vi "Edit Auton Queue Items.vi"(10 "Add?":bool, 11 "Delete?":bool) -> ()   [LabVIEW 2015]
uses:
  Robot Global Data.vi
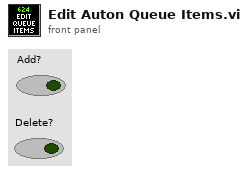
[diagram p1: front panel]
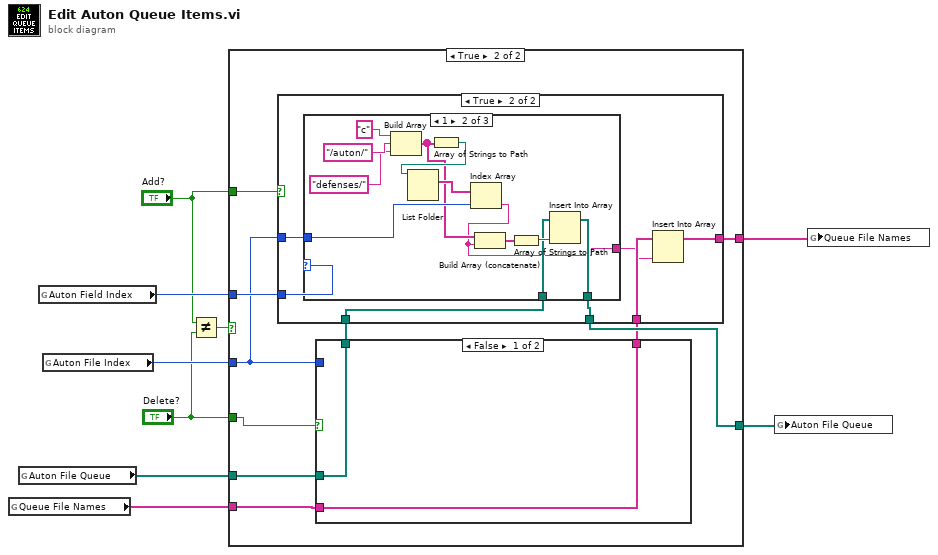
[diagram p0: block diagram]
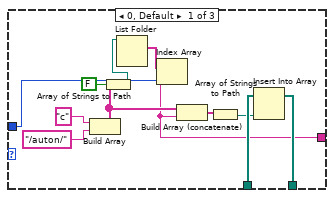
[diagram p4: hidden frame]
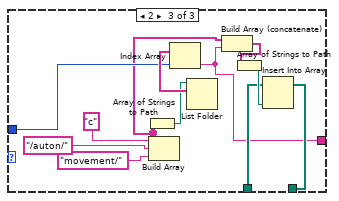
[diagram p5: hidden frame]
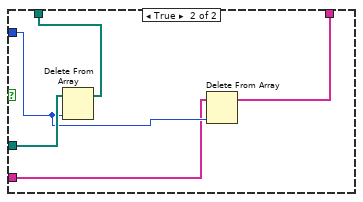
[diagram p6: hidden frame]
diagram:
  n1 = global read "Robot Global Data.vi" "Queue File Names"() -> (w2:string[])
  n2 = global read "Robot Global Data.vi" "Auton File Queue"() -> (w4:path[])
  n3 = global read "Robot Global Data.vi" "Auton Field Index"() -> (w9:i32)
  n4 = global read "Robot Global Data.vi" "Auton File Index"() -> (w8:i32)
  n5 = Not Equal?(x="Add?", y="Delete?") -> (x != y?=w5:bool)
  n6 = case shown="True" w5 {
    tunnel: "Add?" -> [_ w18]
    tunnel: "Delete?" -> [_ w21]
    tunnel: w9 -> [_ w17]
    tunnel: w8 -> [_ w16]
    tunnel: w4 -> [w11 w20]
    tunnel: [w11 w15] -> w3
    tunnel: w2 -> [w10 w14]
    tunnel: [w10 w12] -> w1
    frame False {
    }
    frame True {
      n7 = case shown="False" w21 {
        tunnel: w16 -> [_ w71]
        tunnel: w20 -> [w68 w73]
        tunnel: [w68 w72] -> w19
        tunnel: w14 -> [w67 w70]
        tunnel: [w67 w69] -> w13
        frame False {
        }
        frame True {
          n8 = Delete From Array(array=w73, index=w71) -> (array with subset deleted=w72:path[])  [unwired: 1 in, 1 out]
          n9 = Delete From Array(array=w70, index=w71) -> (array with subset deleted=w69:string[])  [unwired: 1 in, 1 out]
        }
      }
      n10 = case shown="True" w18 {
        tunnel: w19 -> [w23 w28]
        tunnel: w17 -> [_ w30]
        tunnel: w16 -> [_ w29]
        tunnel: [w23 w27] -> w15
        tunnel: w13 -> [w22 w26]
        tunnel: [w22 w24] -> w12
        frame False {
        }
        frame True {
          n11 = case shown="1" w30 {
            tunnel: w29 -> [w42 w52 w63]
            tunnel: w28 -> [w40 w51 w64]
            tunnel: [w38 w50 w62] -> w27
            tunnel: [w31 w43 w55] -> w25
            frame 0, Default {
              n12 = Build Array("c", "/auton/") -> (w33:string[])
              n13 = Array of Strings to Path(0:w33, 1:FALSE ("relative")) -> (2:w35:path)
              n14 = List Folder(path=w35) -> (filenames=w41:string[])  [unwired: 3 in, 3 out]
              n15 = Index Array(array=w41, index=w42) -> (element=w31:string)
              n16 = Build Array (concatenate)(w33, w31) -> (w32:string[])
              n17 = Array of Strings to Path(0:w32) -> (2:w39:path)  [unwired: 1 in]
              n18 = Insert Into Array(array=w40, new element=w39) -> (w38:path[])  [unwired: 1 in]
            }
            frame 1 {
              n19 = Build Array("c", "/auton/", "defenses/" ("element")) -> (w45:string[])
              n20 = Array of Strings to Path(0:w45) -> (2:w47:path)  [unwired: 1 in]
              n21 = List Folder(path=w47) -> (filenames=w53:string[])  [unwired: 3 in, 3 out]
              n22 = Index Array(array=w53, index=w52) -> (element=w43:string)
              n23 = Build Array (concatenate)(w45, w43) -> (w44:string[])
              n24 = Array of Strings to Path(0:w44) -> (2:w54:path)  [unwired: 1 in]
              n25 = Insert Into Array(array=w51, new element=w54) -> (w50:path[])  [unwired: 1 in]
            }
            frame 2 {
              n26 = Build Array("c", "/auton/", "movement/" ("element")) -> (w57:string[])
              n27 = Array of Strings to Path(0:w57) -> (2:w58:path)  [unwired: 1 in]
              n28 = List Folder(path=w58) -> (filenames=w65:string[])  [unwired: 3 in, 3 out]
              n29 = Index Array(array=w65, index=w63) -> (element=w55:string)
              n30 = Build Array (concatenate)(w57, w55) -> (w56:string[])
              n31 = Array of Strings to Path(0:w56) -> (2:w66:path)  [unwired: 1 in]
              n32 = Insert Into Array(array=w64, new element=w66) -> (w62:path[])  [unwired: 1 in]
            }
          }
          n33 = Insert Into Array(array=w26, new element=w25) -> (w24:string[])  [unwired: 1 in]
        }
      }
    }
  }
  n34 = global write "Robot Global Data.vi" "Auton File Queue"(w3) -> ()
  n35 = global write "Robot Global Data.vi" "Queue File Names"(w1) -> ()
